vi "init.vi"(8 "error in (no error)":errorcluster) -> (0 "error out":errorcluster, 3 "Database.lvclass":refnum<class "Account History.lvclass">)   [LabVIEW 2018, in "Account History.lvclass"]
uses:
  Account History.lvclass
  Account History.lvclass/Account History.ctl
  <vilib>/addons/database/Connection.llb/DB Tools Open Connec (String).vi
  <vilib>/addons/database/NI_Database_API.lvlib
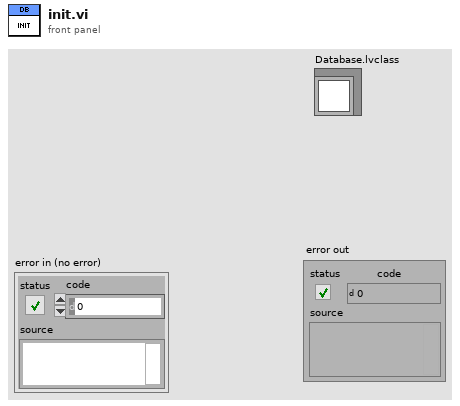
[diagram p1: front panel]
types:
  T1 = typedef "NI_Database_API.lvlib/Conn ObjectReference.ctl" = refnum<k1>
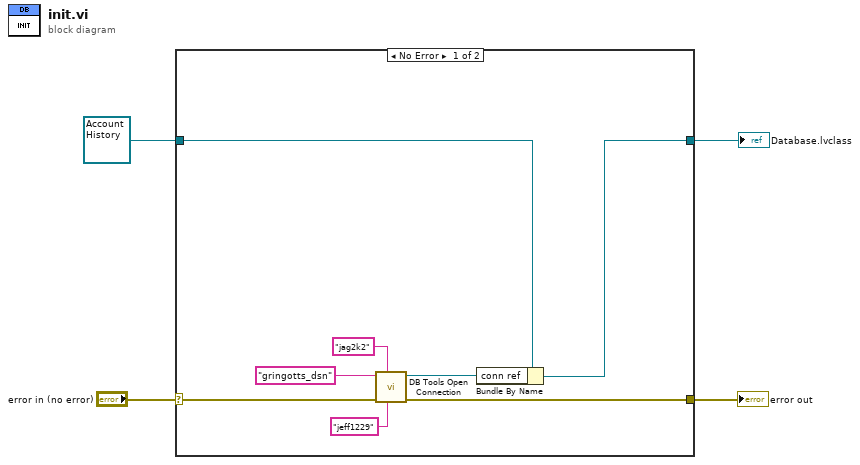
[diagram p0: block diagram]
diagram:
  n1 = case shown="No Error" "error in (no error)" {
    selector: "error in (no error)" -> [w12 w13]
    tunnel: [w11 w13] -> w3
    tunnel: [w9 w14] -> w2
    tunnel: refnum<class "Account History.lvclass"> refnum ("Database.lvclass") -> [w10 w14]
    frame No Error {
      n2 = call-poly <vilib>:"DB Tools Open Connection.vi"("password"="jeff1229", "userID"="jag2k2", "error in (no error)"=w12, "connection information"="gringotts_dsn") -> ("error out"=w11:errorcluster, "connection reference"=w8:T1)  [unwired: 4 in]
      n3 = Bundle By Name(cluster=w10, "conn ref"=w8) -> (w9:refnum<class "Account History.lvclass">)
    }
    frame Error {
    }
  }
  "error out" <- w3
  "Database.lvclass" <- w2
